vi "船舶健康监测.vi"() -> ()   [LabVIEW 2018]
uses:
  <vilib>/Instr/_visa.llb/VISA Configure Serial Port (Instr).vi
  <vilib>/picture/3D Picture Control/Object/Add Object (no reference).vi
  <vilib>/picture/3D Picture Control/NI_3D Picture Control.lvlib
panel:
  in  "VISA资源名称":refnum<visa-resource-name>
  out "?":refnum<vi>(3d-picture)
  out "?":refnum<vi>(3d-picture)
  out "?":refnum<vi>(3d-picture)
  in  "yaw":path caption="3D模型路径"
  out "?":i32(graph)
  out "?":i32(graph)
  out "?":i32(graph)
  out "?":i32(graph)
  out "?":i32(graph)
  in  "baud rate (9600)":u32=9600 caption="波特率"
  out "?":i32(graph)
  out "?":string
  out "下弯超过阈值":bool
  out "上弯超过阈值":bool
  out "原始数据":string
  in  "下阈值":dbl
  in  "上阈值":dbl
  in  "?":bool
  # "船舶健康监测数据显示平台"
  # "功能与使用说明：\n1.应变：实现实时图标显示应变值；阈值报警；周期内统计上传至onenet平台；钉钉机器人报警系统；保存至.txt格式文件。\n\n2.温湿度：实现实时图表显示；保存至.txt文件；\n\n3.姿态：实现实时图表显示；三维动态显示"
  # "应变"
  # "温度"
  # "Roll"
  # "湿度"
  # "Pitch"
  # "阈值\n报警"
  # "写入\n文件\n.txt"
  # "未开发"
  # "串口配置"
  # "Yallh"
  # "未开发"
  # "未开发"
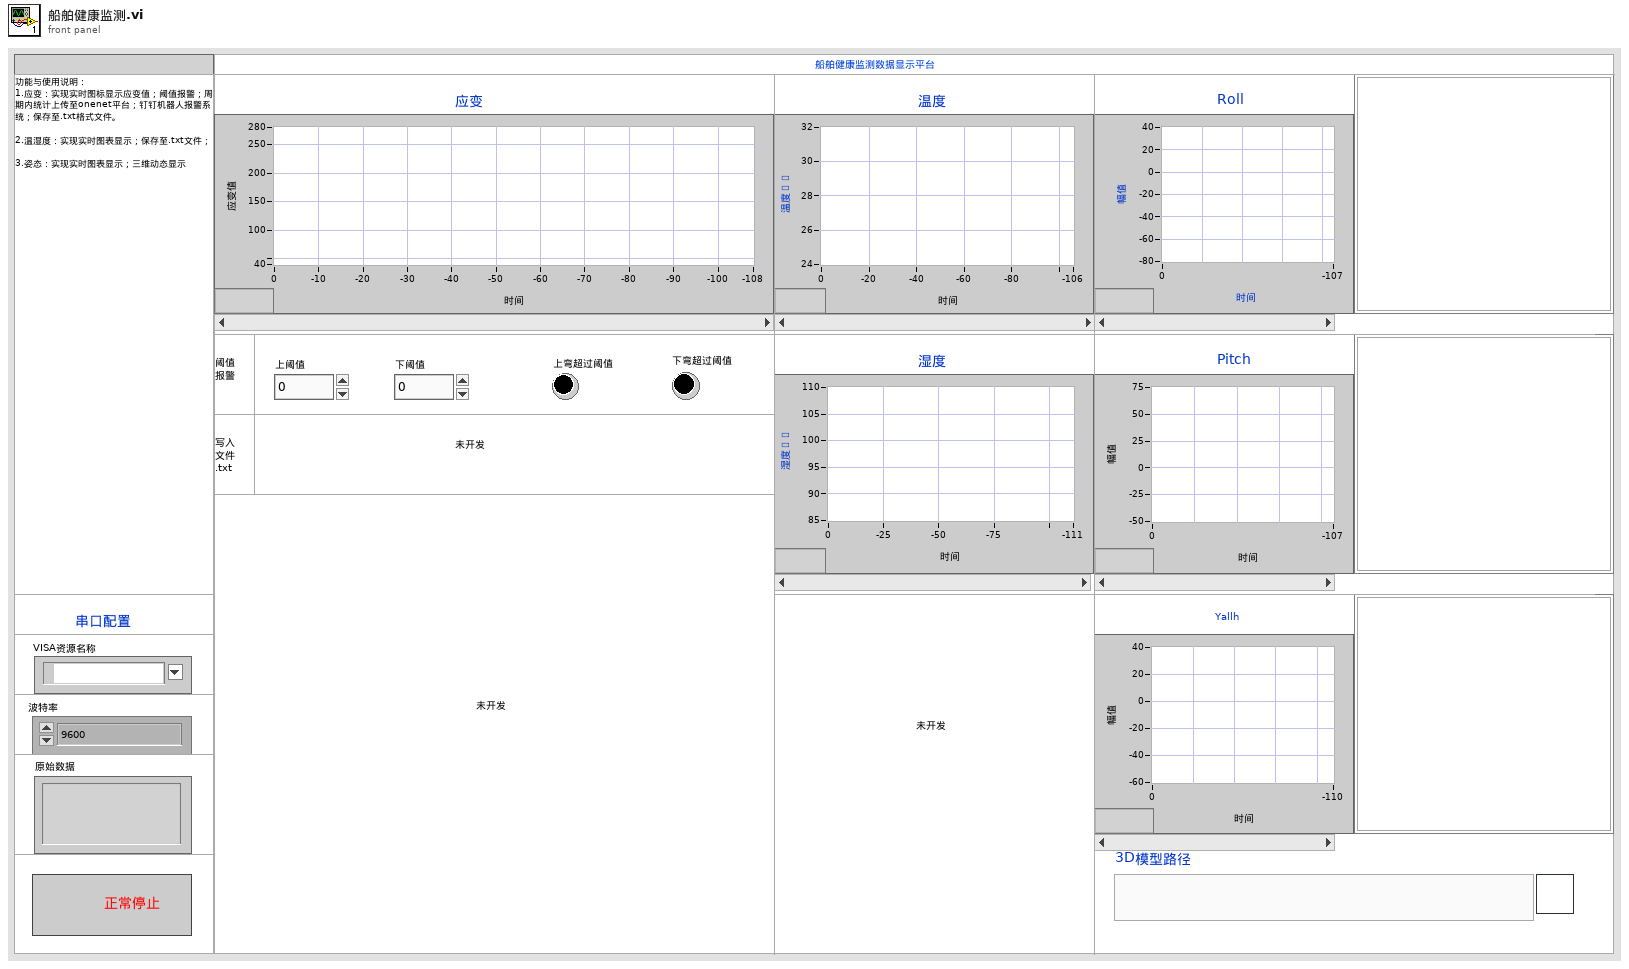
[diagram p1: front panel]
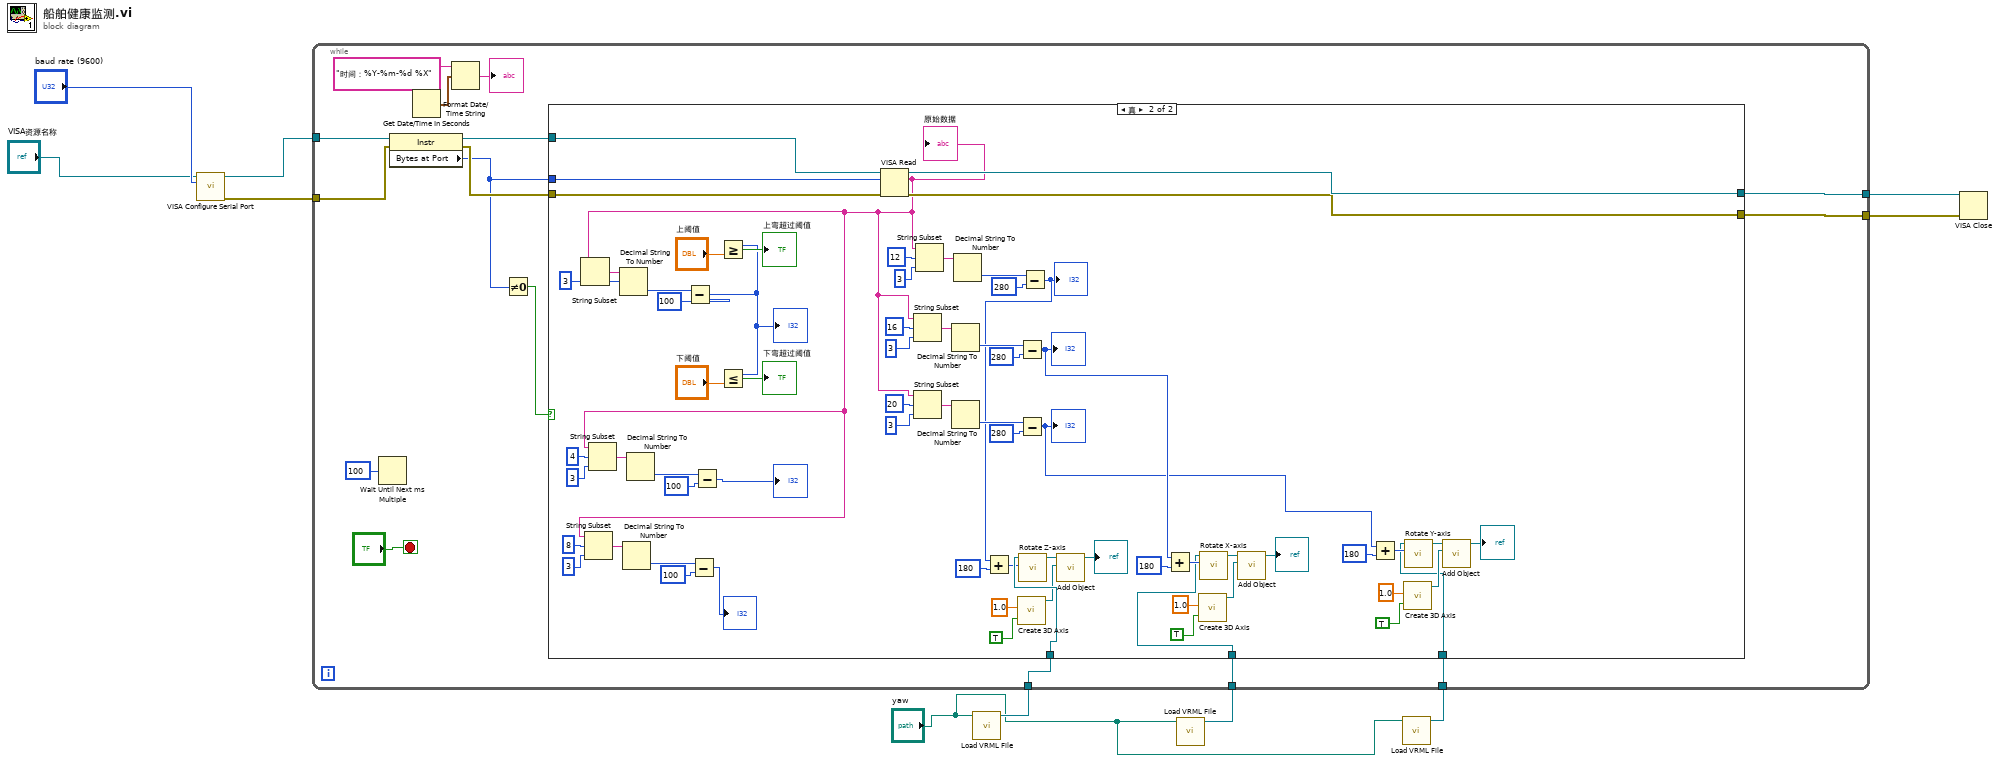
[diagram p0: block diagram]
diagram:
  n1 = call-poly "VISA Configure Serial Port"("VISA resource name"="VISA资源名称", "baud rate (9600)"="baud rate (9600)") -> ("VISA resource name out"=w8:refnum<visa-resource-name>, "error out"=w7:errorcluster)  [unwired: 12 in]
  n2 = call <vilib>:"Load VRML File.vi"("Path"="yaw") -> ("Scene:Read Scene File"=w5:refnum<vi>)  [unwired: 9 in, 1 out]
  n3 = call <vilib>:"Load VRML File.vi"("Path"="yaw") -> ("Scene:Read Scene File"=w4:refnum<vi>)  [unwired: 9 in, 1 out]
  n4 = call <vilib>:"Load VRML File.vi"("Path"="yaw") -> ("Scene:Read Scene File"=w3:refnum<vi>)  [unwired: 9 in, 1 out]
  n5 = while {
    tunnel: w7 -> [w26]
    tunnel: w8 -> [w23]
    tunnel: [w19] -> w10
    tunnel: [w18] -> w9
    tunnel: w5 -> [w13]
    tunnel: w4 -> [w12]
    tunnel: w3 -> [w11]
    stop <- "?" stop-if-true
    n6 = Wait Until Next ms Multiple(millisecond multiple=u32 100 ("毫秒倍数")) -> ()  [unwired: 1 out]
    n7 = property class="Instr"(reference=w23, error in=w26) -> (reference out=w24:refnum<visa-resource-name>, error out=w25:errorcluster, "Bytes at Port"=w22:u32)
    n8 = Get Date/Time In Seconds() -> (seconds since 1Jan1904=w16:timestamp)
    n9 = Format Date/Time String(time format string (%c)="时间：%Y-%m-%d %X", seconds (now)=w16) -> (date/time string=→"?":string)  [unwired: 1 in]
    n10 = Not Equal To 0?(x=w22) -> (x != 0?=w14:bool)
    n11 = case shown="真" w14 {
      tunnel: w25 -> [_ w95]
      tunnel: w24 -> [_ w94]
      tunnel: w22 -> [_ w93]
      tunnel: [_ w92] -> w19
      tunnel: [_ w91] -> w18
      tunnel: w13 -> [_ w53]
      tunnel: w12 -> [_ w30]
      tunnel: w11 -> [_ w28]
      frame False {
      }
      frame True {
        n12 = VISA Read(VISA resource name=w94, byte count=w93, error in (no error)=w95) -> (VISA resource name out=w92:refnum<visa-resource-name>, read buffer=w54:string, error out=w91:errorcluster)  [unwired: 1 out]
        "原始数据" <- w54
        n13 = String Subset(string=w54, length (rest)=3 ("长度（剩余）")) -> (substring=w85:string)  [unwired: 1 in]
        n14 = String Subset(string=w54, offset (0)=8 ("偏移量(0)"), length (rest)=3 ("长度（剩余）")) -> (substring=w82:string)
        n15 = String Subset(string=w54, offset (0)=4 ("偏移量(0)"), length (rest)=3 ("长度（剩余）")) -> (substring=w81:string)
        n16 = Decimal String To Number(string=w85) -> (number=w78:i32)  [unwired: 2 in, 1 out]
        n17 = Decimal String To Number(string=w82) -> (number=w75:i32)  [unwired: 2 in, 1 out]
        n18 = Decimal String To Number(string=w81) -> (number=w72:i32)  [unwired: 2 in, 1 out]
        n19 = Subtract(x=w78, y=100) -> (x-y=w77:i32)
        "?" <- w77
        n20 = Subtract(x=w75, y=100) -> (x-y=→"?":i32)
        n21 = Subtract(x=w72, y=100) -> (x-y=→"?":i32)
        n22 = Greater Or Equal?(x=w77, y="上阈值") -> (x >= y?=→"上弯超过阈值":bool)
        n23 = Less Or Equal?(x=w77, y="下阈值") -> (x <= y?=→"下弯超过阈值":bool)
        n24 = String Subset(string=w54, offset (0)=16 ("偏移量(0)"), length (rest)=3 ("长度（剩余）")) -> (substring=w64:string)
        n25 = String Subset(string=w54, offset (0)=20 ("偏移量(0)"), length (rest)=3 ("长度（剩余）")) -> (substring=w55:string)
        n26 = String Subset(string=w54, offset (0)=12 ("偏移量(0)"), length (rest)=3 ("长度（剩余）")) -> (substring=w65:string)
        n27 = Decimal String To Number(string=w64) -> (number=w61:i32)  [unwired: 2 in, 1 out]
        n28 = Decimal String To Number(string=w55) -> (number=w58:i32)  [unwired: 2 in, 1 out]
        n29 = Decimal String To Number(string=w65) -> (number=w68:i32)  [unwired: 2 in, 1 out]
        n30 = call <vilib>:"Create 3D Axis.vi"("Axis label?"=TRUE, "Length"=sgl 1.0) -> ("New Object Refnum"=w49:refnum<vi>)  [unwired: 8 in, 1 out]
        n31 = Subtract(x=w61, y=280) -> (x-y=w29:i32)
        "?" <- w29
        n32 = Subtract(x=w58, y=280) -> (x-y=w27:i32)
        "?" <- w27
        n33 = Subtract(x=w68, y=280) -> (x-y=w47:i32)
        "?" <- w47
        n34 = Add(x=w47, y=180) -> (x+y=w46:i32)
        n35 = call <vilib>:"Rotate Z-axis.vi"("angle"=w46, "Scene Object In"=w53) -> ("Scene Object Out"=w50:refnum<vi>)  [unwired: 8 in, 1 out]
        n36 = call-poly <vilib>:"Add Object.vi"("New Object In"=w49, "Scene Object In"=w50) -> ("Scene Object Out"=→"?":refnum<vi>)  [unwired: 8 in, 1 out]
        n37 = Add(x=w29, y=180) -> (x+y=w43:i32)
        n38 = call <vilib>:"Create 3D Axis.vi"("Axis label?"=TRUE, "Length"=sgl 1.0) -> ("New Object Refnum"=w41:refnum<vi>)  [unwired: 8 in, 1 out]
        n39 = call <vilib>:"Rotate X-axis.vi"("angle"=w43, "Scene Object In"=w30) -> ("Scene Object Out"=w40:refnum<vi>)  [unwired: 8 in, 1 out]
        n40 = call-poly <vilib>:"Add Object.vi"("New Object In"=w41, "Scene Object In"=w40) -> ("Scene Object Out"=→"?":refnum<vi>)  [unwired: 8 in, 1 out]
        n41 = Add(x=w27, y=180) -> (x+y=w32:i32)
        n42 = call <vilib>:"Create 3D Axis.vi"("Axis label?"=TRUE, "Length"=sgl 1.0) -> ("New Object Refnum"=w34:refnum<vi>)  [unwired: 8 in, 1 out]
        n43 = call <vilib>:"Rotate Y-axis.vi"("angle"=w32, "Scene Object In"=w28) -> ("Scene Object Out"=w35:refnum<vi>)  [unwired: 8 in, 1 out]
        n44 = call-poly <vilib>:"Add Object.vi"("New Object In"=w34, "Scene Object In"=w35) -> ("Scene Object Out"=→"?":refnum<vi>)  [unwired: 8 in, 1 out]
      }
    }
  }
  n45 = VISA Close(VISA resource name=w10, error in (no error)=w9) -> ()  [unwired: 1 out]
